vi "read state.vi"(8 "error in (no error)":errorcluster, 11 "PSP-603 in":refnum<class "PSP-603.lvclass">) -> (0 "error out":errorcluster, 2 "Variant":variant, 3 "PSP-603 out":refnum<class "PSP-603.lvclass">)   [LabVIEW 2025, in "Power Supply.lvlib" / "PSP-603.lvclass"]
uses:
  PSP-603.lvclass
  PSP-603.lvclass/PSP-603.ctl
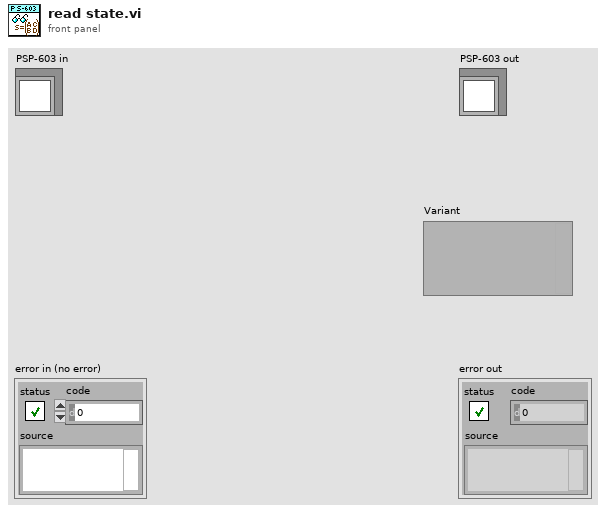
[diagram p1: front panel]
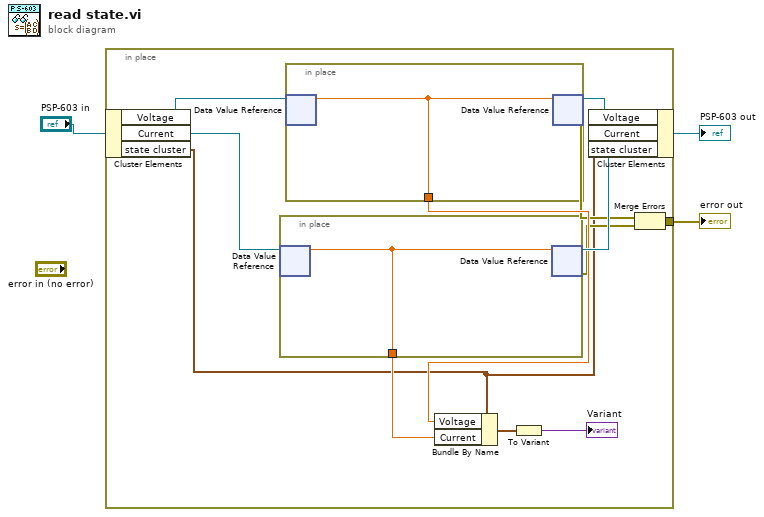
[diagram p0: block diagram]
diagram:
  n1 = in-place {
    in-place-border: [w5] -> w1
    n2 = in-place-cluster #1("PSP-603 in") -> ("Voltage"=w15:refnum<data-value>, "Current"=w14:refnum<data-value>, "state cluster"=w4:cluster{"Voltage":dbl, "Current":dbl})
    n3 = in-place {
      in-place-border: [w16] -> w10
      n4 = in-place-dvr #2(w14) -> (w16:dbl)  [unwired: 1 out]
      n5 = in-place-dvr #2(w16) -> (w12:refnum<data-value>, w7:errorcluster)
    }
    n6 = in-place {
      in-place-border: [w17] -> w11
      n7 = in-place-dvr #3(w15) -> (w17:dbl)  [unwired: 1 out]
      n8 = in-place-dvr #3(w17) -> (w13:refnum<data-value>, w6:errorcluster)
    }
    n9 = Bundle By Name(cluster=w4, "Voltage"=w11, "Current"=w10) -> (w9:cluster{"Voltage":dbl, "Current":dbl})
    n10 = To Variant(anything=w9) -> (Variant=→"Variant":variant)
    n11 = in-place-cluster #1("Voltage"=w13, "Current"=w12, "state cluster"=w4) -> (→"PSP-603 out":refnum<class "PSP-603.lvclass">)
    n12 = Merge Errors(w6, w7) -> (w5:errorcluster)
  }
  "error out" <- w1
